vi "Shutdown.vi"(8 "error in":errorcluster, 11 "PowerSupply in":refnum<class "PowerSupply.lvclass">) -> (0 "error out":errorcluster, 3 "PowerSupply out":refnum<class "PowerSupply.lvclass">)   [LabVIEW 2019, in "PowerSupply.lvlib" / "PowerSupply.lvclass"]
uses:
  Library/PowerSupply.lvclass
  builds/Instruments/Instruments.lvlibp/Library/Instruments.lvclass
  builds/Engine/Engine.lvlibp/Project/Engine.lvclass
  C:/Users/Public/Documents/Development/builds/Instruments/Instruments.lvlibp/Library/Instruments.lvclass
  C:/Users/Public/Documents/Development/builds/Tools/Config.lvlibp/Config.lvclass
  C:/Users/Public/Documents/Development/builds/Engine/Engine.lvlibp/Project/Engine.lvclass
  C:/Users/Public/Documents/Development/builds/Engine/State Actor.lvlibp/Library/State Actor.lvclass
  C:/Users/Public/Documents/Development/builds/Engine/Panel Manager.lvlibp/Panel Actor/Panel Actor.lvclass
  C:/Users/Public/Documents/Development/builds/Engine/Monitored Actor.lvlibp/Monitored Actor/Monitored Actor/Monitored Actor.lvclass
  C:/Users/Public/Documents/Development/builds/Engine/Actor Framework.lvlibp/1abvi3w/vi.lib/ActorFramework/Actor/Actor.lvclass
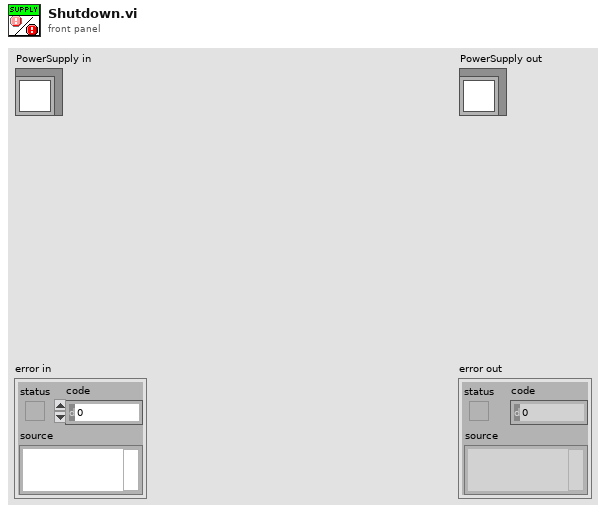
[diagram p1: front panel]
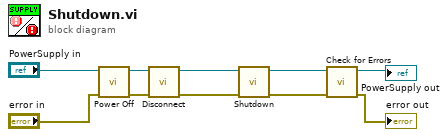
[diagram p0: block diagram]
diagram:
  n1 = call-dynamic "Power Off.vi"("error in"="error in", "PowerSupply in"="PowerSupply in") -> ("error out"=w1:errorcluster, "PowerSupply out"=w3:refnum<class "PowerSupply.lvclass">)  [unwired: 8 in]
  n2 = call-dynamic "Disconnect.vi"("error in"=w1, "PowerSupply in"=w3) -> ("error out"=w5:errorcluster, "PowerSupply out"=w8:refnum<class "PowerSupply.lvclass">)  [unwired: 8 in]
  n3 = call-parent "Shutdown.vi"("error in"=w5, "Instruments in"=w8) -> ("error out"=w6:errorcluster, "Instruments out"=w7:refnum<class "PowerSupply.lvclass">)  [unwired: 8 in]
  n4 = call "Check for Errors.vi"("error in"=w6, "Engine in"=w7) -> ("error out"=→"error out":errorcluster, "Engine out"=→"PowerSupply out":refnum<class "PowerSupply.lvclass">)  [unwired: 8 in]
